vi "Creators Status Created Events.vi"(11 "Hello World Event in":refnum<class "Hello World Event.lvclass">) -> (0 "Created Event Count":i32, 1 "Created Event Aliases":string[](array[string]), 2 "Created Event Exist?":bool, 3 "Hello World Event out":refnum<class "Hello World Event.lvclass">)   [LabVIEW 2021, in "Hello World Event.lvlib" / "Hello World Event.lvclass"]
uses:
  Hello World Event.lvclass
  Hello World Event.lvclass/Hello World Event.ctl
  jettl/Event jettl/Event jettl.lvclass
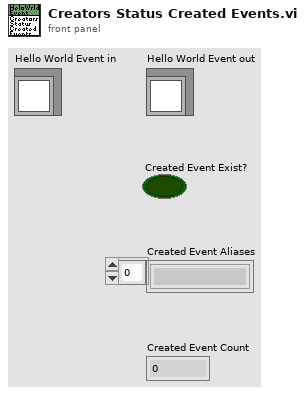
[diagram p1: front panel]
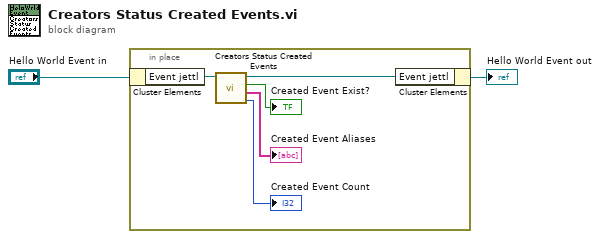
[diagram p0: block diagram]
diagram:
  n1 = in-place {
    n2 = in-place-cluster #1("Hello World Event in") -> ("Event jettl"=w7:refnum<class "Event jettl.lvclass">)
    n3 = call-dynamic "Creators Status Created Events.vi"("Event jettl in"=w7) -> ("Created Event Count"=→"Created Event Count":i32, "Created Event Aliases"=→"Created Event Aliases":string[], "Created Event Exist?"=→"Created Event Exist?":bool, "Event jettl out"=w6:refnum<class "Event jettl.lvclass">)  [unwired: 7 in]
    n4 = in-place-cluster #1("Event jettl"=w6) -> (→"Hello World Event out":refnum<class "Hello World Event.lvclass">)
  }
